vi "addMixtureDensity.vi"(0 "error in (no error) 2":errorcluster, 1 "ptr":i64, 2 "Mixture Coefficients (K)":u32, 3 "NOUT (L)":u32, 4 "Blocks":u32) -> (5 "error in (no error)":errorcluster, 6 "ptr out":i64)   [LabVIEW 2016, in "CNet.lvlib"]
uses:
  CNet.lvlib
  Users/jg754/Documents/Visual Studio 2015/Projects/CLearn/x64/Release/CLearn.dll
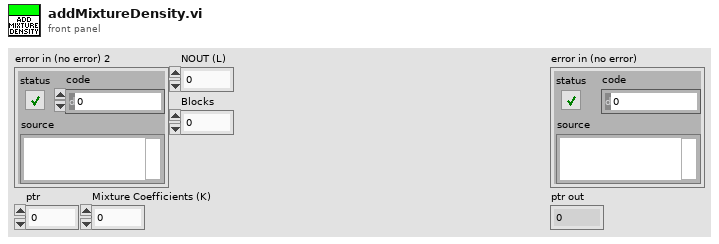
[diagram p1: front panel]
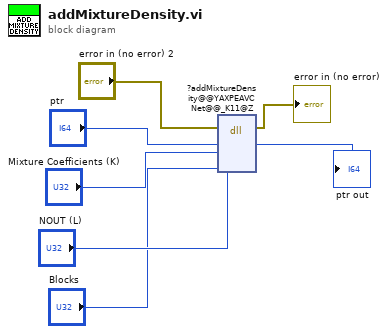
[diagram p0: block diagram]
diagram:
  n1 = dll-call lib="C:/Users/jg754/Documents/Visual Studio 2015/Projects/CLearn/x64/Release/CLearn.dll" fn="?addMixtureDensity@@YAXPEAVCNet@@_K11@Z"(error in="error in (no error) 2", "ptr"="ptr", "Mixture Coefficients (K)"="Mixture Coefficients (K)", "NOUT (L)"="NOUT (L)", "Blocks"="Blocks") -> (error out=→"error in (no error)":errorcluster, "ptr"=→"ptr out":i64)  [unwired: 6 in, 1 out]
